vi "Release All.vi"(8 "error in (no error)":errorcluster, 11 "Available Handles":u64[](array[numeric])) -> (0 "error out":errorcluster)   [LabVIEW 2012, in "Phidget Manager.lvlib"]
doc: "Cleans up after List Available Phidgets.vi"
uses:
  <instrlib>/Phidgets/Phidget Manager/Phidget Manager.lvlib
  <instrlib>/Phidgets/Phidget Common/Phidget Common.lvlib
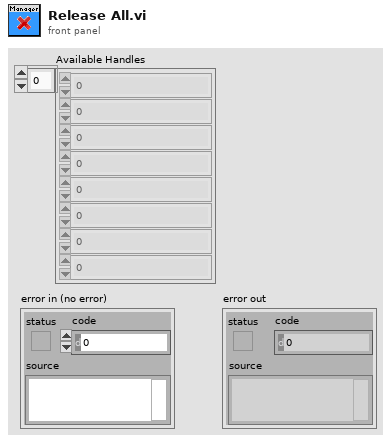
[diagram p1: front panel]
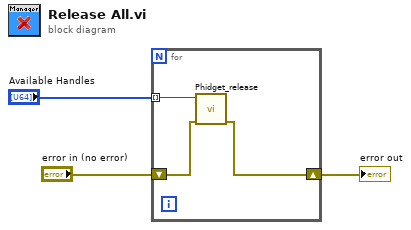
[diagram p0: block diagram]
diagram:
  n1 = for {
    tunnel: "Available Handles" -> [w6] mode=indexing
    shift-right: [w4] -> w1
    shift-left: "error in (no error)" -> [w5]
    n2 = call <instrlib>:"Phidget_release.vi"("error in"=w5, "Device In"=w6) -> ("error out"=w4:errorcluster)  [unwired: 9 in]
  }
  "error out" <- w1
